vi "Log Data_PID.vi"(0 "refnum in":refnum<file>, 1 "Temp (C)":dbl, 2 "Heater Status":bool, 3 "Set Point FB":i32 caption="Temp Set Point (C)", 4 "On/Off Set":bool, 5 "Error In":errorcluster, 7 "PID values":dbl[](array[numeric]), 9 "PWM":i32) -> (14 "refnum out":refnum<file>, 19 "Error Out":errorcluster)   [LabVIEW 2015]
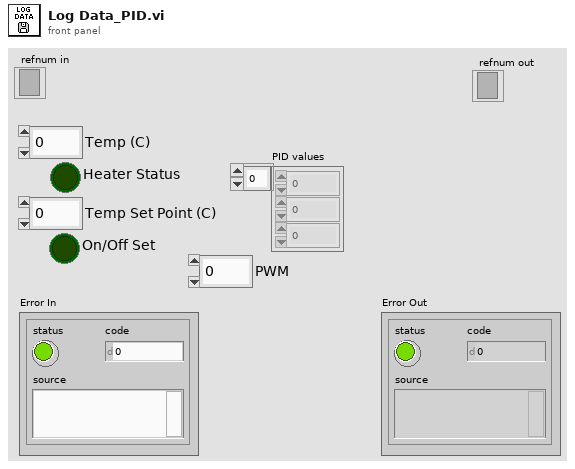
[diagram p1: front panel]
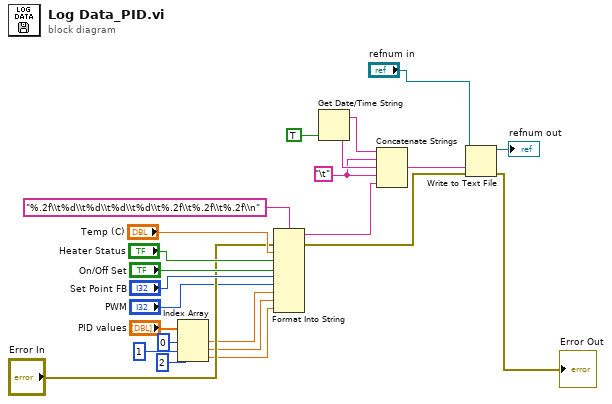
[diagram p0: block diagram]
diagram:
  w20 = "\t"
  n1 = Index Array(array="PID values", index #1=0 ("index"), index #2=1 ("index"), index #3=2 ("index")) -> (element #1=w2:dbl, element #2=w3:dbl, element #3=w4:dbl)
  n2 = Format Into String(format string="%.2f\\t%d\\t%d\\t%d\\t%d\\t%.2f\\t%.2f\\t%.2f\\n", error in="Error In", "Temp (C)", "Heater Status", "On/Off Set", "Set Point FB", "PWM", w2, w3, w4) -> (resulting string=w15:string, error out=w10:errorcluster)  [unwired: 1 in]
  n3 = Get Date/Time String(want seconds? (F)=TRUE) -> (date string=w23:string, time string=w22:string)  [unwired: 2 in]
  n4 = Concatenate Strings(w23, w20, w22, w20, w15) -> (w21:string)
  n5 = Write to Text File(file (use dialog)="refnum in", text=w21, error in=w10) -> (refnum out=→"refnum out":refnum<file>, error out=→"Error Out":errorcluster)  [unwired: 1 in, 1 out]
